vi "MATRIX.vi"() -> ()   [LabVIEW 2012]
uses:
  <vilib>/Instr/_visa.llb/VISA Configure Serial Port (Instr).vi
panel:
  in  "Texte":string
  in  "Afficher":bool
  in  "Effacer":bool
  in  "Défilement 2":bool
  in  "Afficher l'heure":bool
  in  "Envoyer un texte":bool
  out "Array booleano":bool[][](array[boolean])
  in  "Colonnes":u32=30
  in  "Texte d'éssai":string
  in  "Défilement":bool
  in  "Abrir fuente":bool
  in  "Salir":bool
  in  "Vitesse de défilement":dbl(slide)=21.09090909090909 scale=1.0..40.0
  out "chaîne d'heure":string
  out "chaîne de date":string
  out "Date et heure":timestamp format="%<%X\n%x>T"
  in  "COM Port":refnum<visa-resource-name>
  # "Mini Projet 2015"
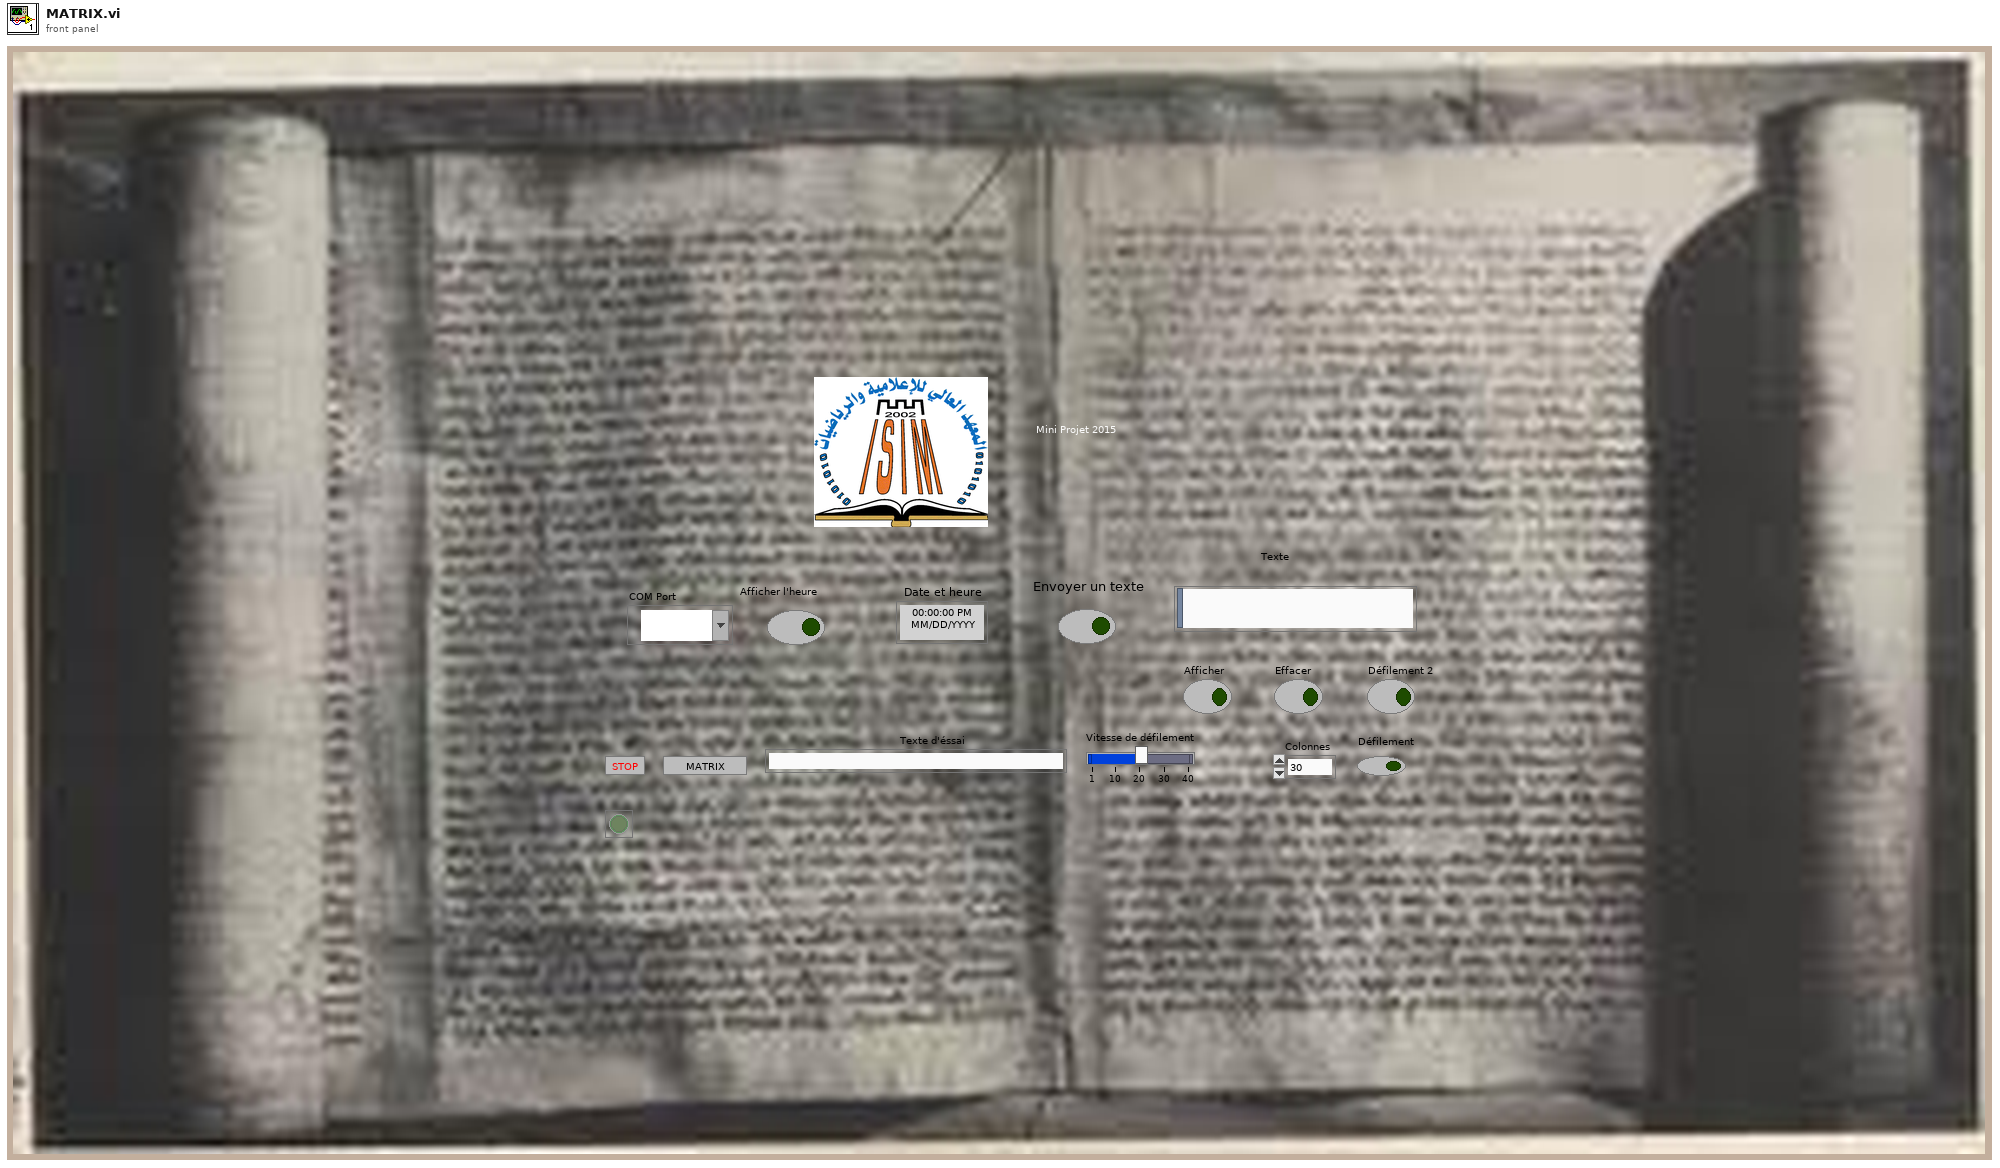
[diagram p1: front panel]
types:
  T1 = enum16{"open", "replace", "create", "open or create", "replace or create", "replace or create with confirmation"}
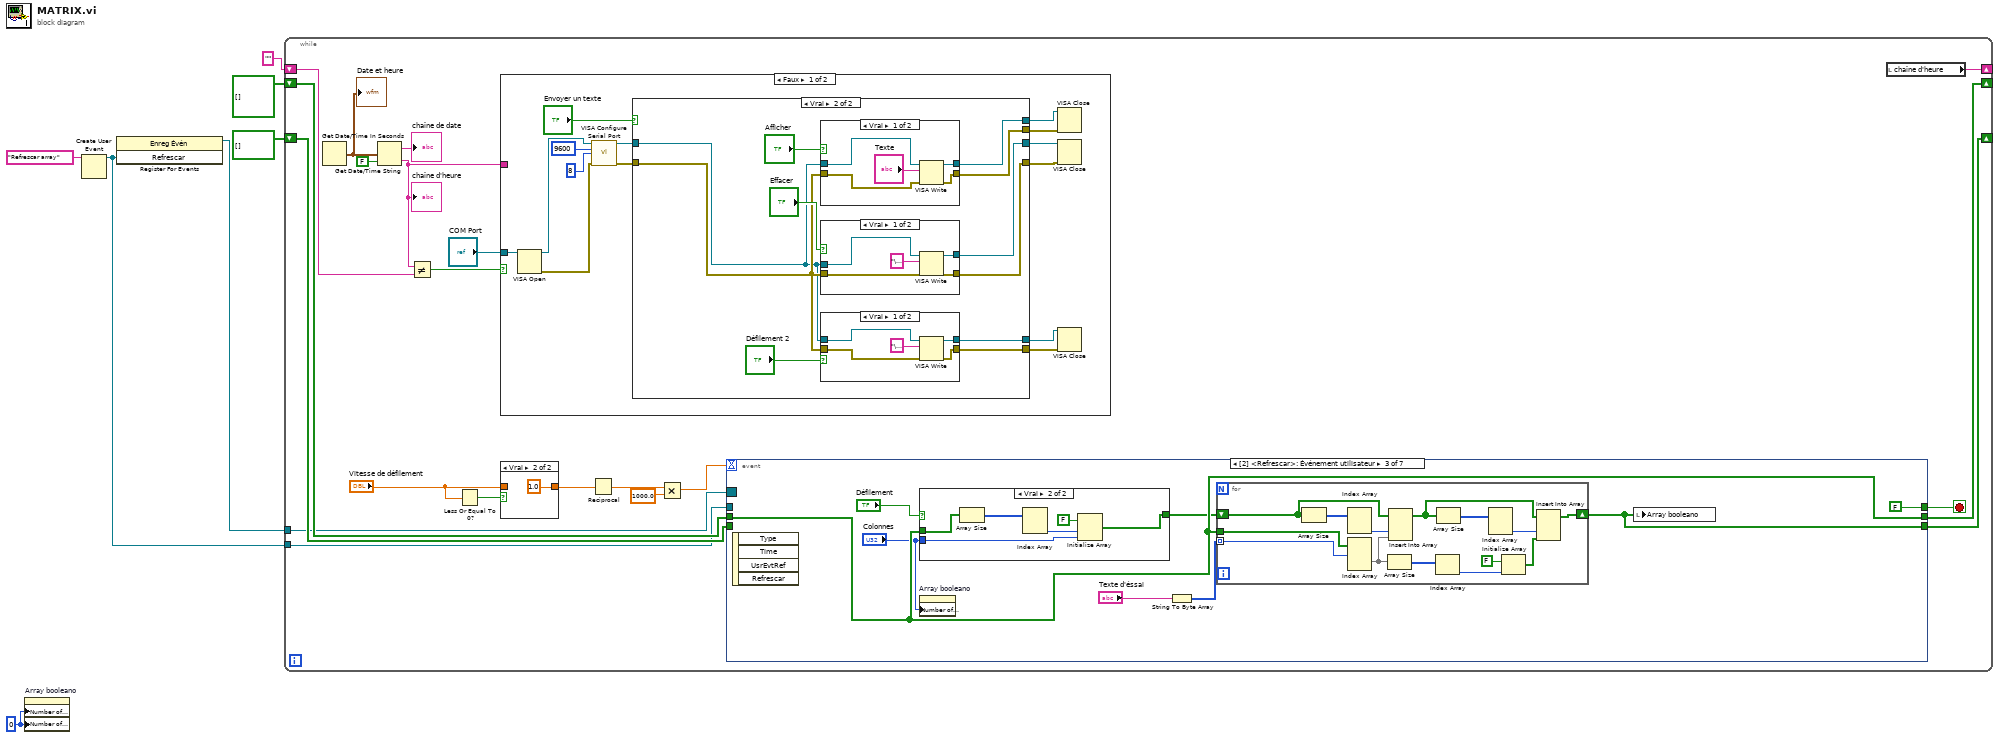
[diagram p0: block diagram]
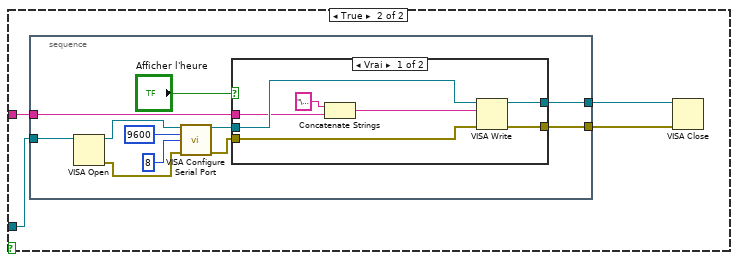
[diagram p6: hidden frame]
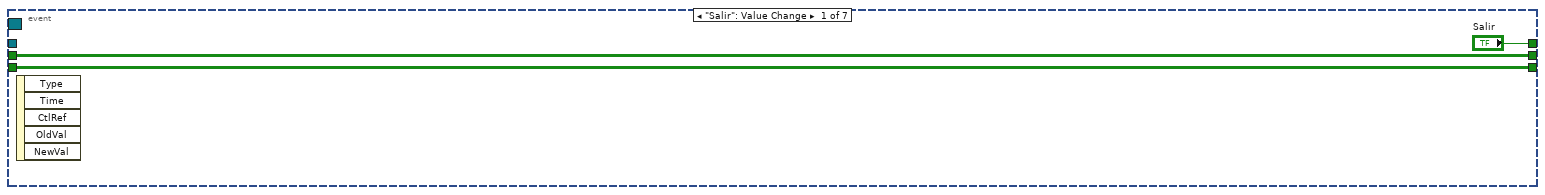
[diagram p9: hidden frame]
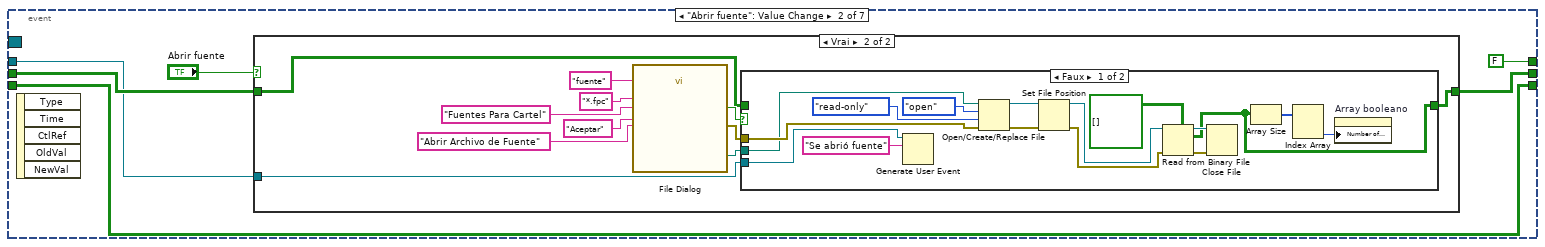
[diagram p10: hidden frame]
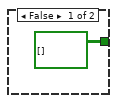
[diagram p13: hidden frame]
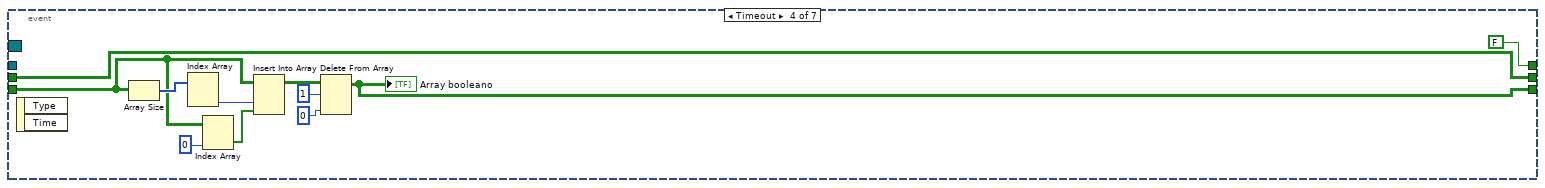
[diagram p14: hidden frame]
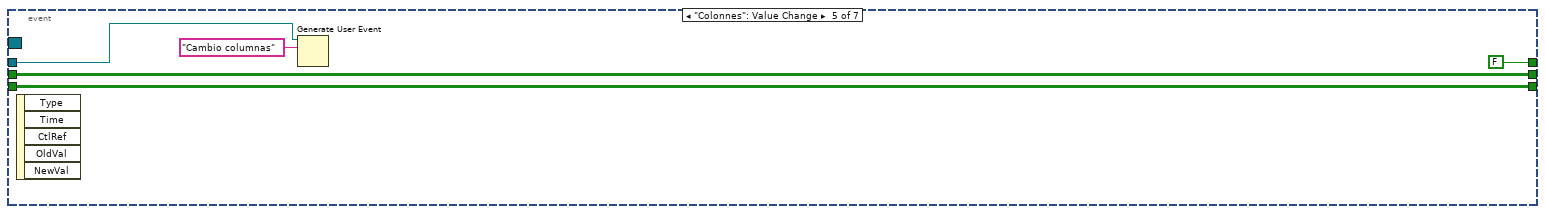
[diagram p15: hidden frame]
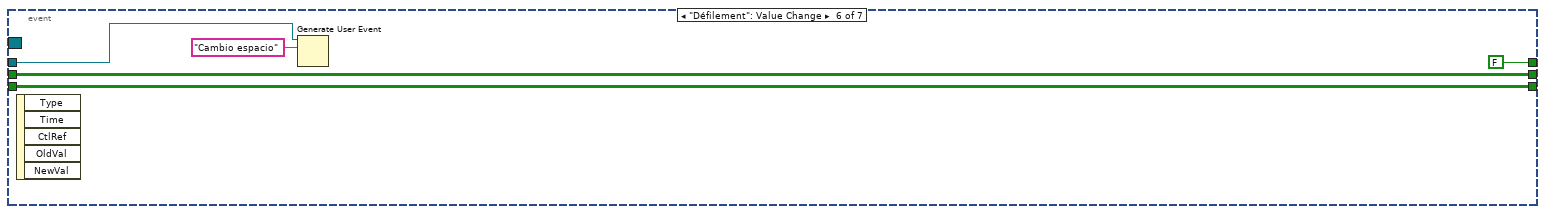
[diagram p16: hidden frame]
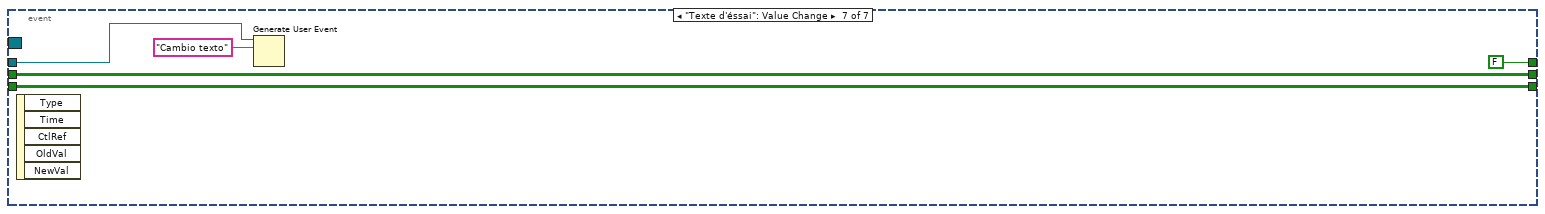
[diagram p17: hidden frame]
diagram:
  w2 = u32 0 ("Number of Columns")
  n1 = property on="Array booleano" class="Tabl (strict)"("Number of Columns"=w2, "Number of Rows"=w2) -> ()  [unwired: 2 in, 2 out]
  n2 = Create User Event(user event datatype="Refrescar array" ("Refrescar")) -> (user event=w3:refnum<user-event>)  [unwired: 1 in, 1 out]
  n3 = register-events(w3) -> (reference out=w4:refnum<event-registration>)  [unwired: 2 in, 1 out]
  n4 = while {
    shift-right: [w20] -> _
    shift-left: bool[][][] [] ("appended array") -> [w19]
    shift-right: [w21] -> _
    shift-left: bool[][] [] ("Array booleano") -> [w18]
    tunnel: w4 -> [w17]
    tunnel: w3 -> [w16]
    shift-right: [w11] -> _
    shift-left: "" ("chaîne d'heure") -> [w9]
    stop <- w15 stop-if-true
    n5 = Get Date/Time In Seconds() -> (seconds since 1Jan1904=w12:timestamp)
    "Date et heure" <- w12
    n6 = Get Date/Time String(seconds (now)=w12, want seconds? (F)=FALSE ("secondes ? (F)")) -> (date string=→"chaîne de date":string, time string=w10:string)  [unwired: 1 in]
    "chaîne d'heure" <- w10
    n7 = Not Equal?(x=w10, y=w9) -> (x != y?=w8:bool)
    n8 = Less Or Equal To 0?(x="Vitesse de défilement") -> (x <= 0?=w24:bool)
    n9 = case shown="Faux" w8 {
      tunnel: "COM Port" -> [w38 w80]
      tunnel: w10 -> [_ w77]
      frame False {
        n10 = VISA Open(VISA resource name=w38) -> (VISA resource name=w40:refnum<visa-resource-name>, error out=w39:errorcluster)  [unwired: 4 in]
        n11 = call-poly "VISA Configure Serial Port"("VISA resource name"=w40, "baud rate (9600)"=u32 9600, "data bits (8)"=u16 8, "error in (no error)"=w39) -> ("VISA resource name out"=w36:refnum<visa-resource-name>, "error out"=w37:errorcluster)  [unwired: 10 in]
        n12 = case shown="Vrai" "Envoyer un texte" {
          tunnel: [w44 w54] -> w30
          tunnel: [w43 w53] -> w29
          tunnel: [w44 w52] -> w32
          tunnel: [w43 w51] -> w31
          tunnel: w37 -> [w43 w48]
          tunnel: w36 -> [w44 w47]
          tunnel: [w44 w46] -> w34
          tunnel: [w43 w45] -> w33
          frame False {
          }
          frame True {
            n13 = case shown="Vrai" "Afficher" {
              tunnel: w48 -> [w74 w75]
              tunnel: w47 -> [w73 w76]
              tunnel: [w72 w76] -> w54
              tunnel: [w71 w75] -> w53
              frame True {
                n14 = VISA Write(VISA resource name=w73, write buffer="Texte", error in (no error)=w74) -> (VISA resource name out=w72:refnum<visa-resource-name>, error out=w71:errorcluster)  [unwired: 1 out]
              }
              frame False {
              }
            }
            n15 = case shown="Vrai" "Effacer" {
              tunnel: w48 -> [w67 w68]
              tunnel: w47 -> [w66 w69]
              tunnel: [w65 w69] -> w52
              tunnel: [w64 w68] -> w51
              frame True {
                n16 = VISA Write(VISA resource name=w66, write buffer="\u0004" ("buffer d'écriture"), error in (no error)=w67) -> (VISA resource name out=w65:refnum<visa-resource-name>, error out=w64:errorcluster)  [unwired: 1 out]
              }
              frame False {
              }
            }
            n17 = case shown="Vrai" "Défilement 2" {
              tunnel: w48 -> [w60 w61]
              tunnel: w47 -> [w59 w62]
              tunnel: [w58 w62] -> w46
              tunnel: [w57 w61] -> w45
              frame True {
                n18 = VISA Write(VISA resource name=w59, write buffer="\u000b" ("buffer d'écriture"), error in (no error)=w60) -> (VISA resource name out=w58:refnum<visa-resource-name>, error out=w57:errorcluster)  [unwired: 1 out]
              }
              frame False {
              }
            }
          }
        }
        n19 = VISA Close(VISA resource name=w30, error in (no error)=w29) -> ()  [unwired: 1 out]
        n20 = VISA Close(VISA resource name=w32, error in (no error)=w31) -> ()  [unwired: 1 out]
        n21 = VISA Close(VISA resource name=w34, error in (no error)=w33) -> ()  [unwired: 1 out]
      }
      frame True {
        n22 = stacked-sequence {
          tunnel: w80 -> [w89]
          tunnel: [w87] -> w79
          tunnel: [w88] -> w78
          tunnel: w77 -> [w82]
          frame #0 {
            n23 = VISA Open(VISA resource name=w89) -> (VISA resource name=w90:refnum<visa-resource-name>, error out=w91:errorcluster)  [unwired: 4 in]
            n24 = call-poly "VISA Configure Serial Port"("VISA resource name"=w90, "baud rate (9600)"=u32 9600, "data bits (8)"=u16 8, "error in (no error)"=w91) -> ("VISA resource name out"=w83:refnum<visa-resource-name>, "error out"=w84:errorcluster)  [unwired: 10 in]
            n25 = case shown="Vrai" "Afficher l'heure" {
              tunnel: w84 -> [w98 w99]
              tunnel: w83 -> [w97 w100]
              tunnel: [w96 w100] -> w88
              tunnel: [w95 w99] -> w87
              tunnel: w82 -> [w94 _]
              frame True {
                n26 = Concatenate Strings("\u0004" ("chaîne"), w94) -> (w93:string)
                n27 = VISA Write(VISA resource name=w97, write buffer=w93, error in (no error)=w98) -> (VISA resource name out=w96:refnum<visa-resource-name>, error out=w95:errorcluster)  [unwired: 1 out]
              }
              frame False {
              }
            }
          }
        }
        n28 = VISA Close(VISA resource name=w78, error in (no error)=w79) -> ()  [unwired: 1 out]
      }
    }
    n29 = case shown="Vrai" w24 {
      tunnel: "Vitesse de défilement" -> [w101 _]
      tunnel: [w101 1.0 ("Velocidad texto [caracteres/segundo]")] -> w25
      frame False {
      }
      frame True {
      }
    }
    n30 = Reciprocal(x=w25) -> (1/x=w26:dbl)
    n31 = Multiply(x=w26, y=1000.0) -> (x*y=w22:dbl)
    n32 = event shown="[2] <Refrescar>: Événement utilisateur" {
      selector: w17 -> [_ _ _ _ _ _ _]
      dyn-events: _ -> [_ _ _ _ _ _ _]
      timeout: w22 -> [_ _ _ _ _ _ _]
      tunnel: ["Salir" FALSE ("Salir") FALSE ("Salir") FALSE ("Salir") FALSE ("Salir") FALSE ("Salir") FALSE ("Salir")] -> w15
      tunnel: w19 -> [w104 w109 w143 w179 w184 w187 w192]
      tunnel: [w104 w108 w143 w179 w184 w187 w192] -> w20
      tunnel: w16 -> [_ w107 _ _ w183 w189 w194]
      tunnel: w18 -> [w103 w106 _ w177 w181 w188 w193]
      tunnel: [w103 w106 w145 w173 w181 w188 w193] -> w21
      event "Salir": Value Change {
        n33 = event-data() -> ()  [unwired: 1 in, 5 out]
      }
      event "Abrir fuente": Value Change {
        n34 = event-data() -> ()  [unwired: 1 in, 5 out]
        n35 = case shown="Vrai" "Abrir fuente" {
          tunnel: [w112 w115] -> w108
          tunnel: w109 -> [w112 w114]
          tunnel: w107 -> [_ w113]
          frame False {
          }
          frame True {
            n36 = call "File Dialog"("prompt"="Abrir Archivo de Fuente", "button label"="Aceptar", "default name"="fuente", "pattern (all files)"="*.fpc", "pattern label"="Fuentes Para Cartel") -> ("selected path"=w116:path, "cancelled"=w118:bool, "error out"=w117:errorcluster)  [unwired: 7 in, 1 out]
            n37 = case shown="Faux" w118 {
              tunnel: w117 -> [w139 _]
              tunnel: w116 -> [w129 _]
              tunnel: [w128 w140] -> w115
              tunnel: w114 -> [_ w140]
              tunnel: w113 -> [w125 _]
              frame False {
                n38 = Generate User Event(user event=w125, event data cluster="Se abrió fuente" ("event data")) -> ()  [unwired: 1 in, 2 out]
                n39 = Open/Create/Replace File(file path (use dialog)=w129, error in=w139, operation (0:open)=T1."open", access (0:read/write)=enum16{"read/write", "read-only", "write-only"}."read-only") -> (refnum out=w135:refnum<file>, error out=w136:errorcluster)  [unwired: 2 in, 1 out]
                n40 = Set File Position(refnum=w135, error in=w136) -> (refnum out=w133:refnum<file>, error out=w134:errorcluster)  [unwired: 2 in]
                n41 = Read from Binary File(5:bool[][][] [] ("appended array"), 8:w134, 11:w133) -> (0:w131:errorcluster, 2:w128:bool[][][], 3:w132:refnum<file>)  [unwired: 3 in, 1 out]
                n42 = Close File(refnum=w132, error in=w131) -> ()  [unwired: 2 out]
                n43 = Array Size(array=w128) -> (size(s)=w127:i32[])
                n44 = Index Array(array=w127) -> (element #2=w126:i32)  [unwired: 2 in, 1 out]
                n45 = property on="Array booleano" class="Tabl (strict)"("Number of Rows"=w126) -> ()  [unwired: 2 in, 2 out]
              }
              frame True {
              }
            }
          }
        }
      }
      event User Event {
        n46 = event-data() -> ()  [unwired: 1 in, 4 out]
        n47 = case shown="Vrai" "Défilement" {
          tunnel: w143 -> [_ w153]
          tunnel: "Colonnes" -> [_ w151]
          tunnel: [bool[][] [] ("Array booleano") w150] -> w141
          frame False {
          }
          frame True {
            n48 = Array Size(array=w153) -> (size(s)=w155:i32[])
            n49 = Index Array(array=w155) -> (element #2=w152:i32)  [unwired: 2 in, 1 out]
            n50 = Initialize Array(FALSE, w152, w151) -> (w150:bool[][])
          }
        }
        n51 = property on="Array booleano" class="Tabl (strict)"("Number of Columns"="Colonnes") -> ()  [unwired: 2 in, 2 out]
        n52 = String To Byte Array(string="Texte d'éssai") -> (unsigned byte array=w146:u8[])
        n53 = for {
          tunnel: w146 -> [w168] mode=indexing
          shift-right: [w163] -> w145
          shift-left: w141 -> [w167]
          tunnel: w143 -> [w169]
          n54 = Array Size(array=w167) -> (size(s)=w166:i32[])
          n55 = Index Array(array=w166) -> (element #2=w156:i32)  [unwired: 2 in, 1 out]
          n56 = Index Array(array=w169, index (dim 0)=w168) -> (element=w162:bool[][])  [unwired: 2 in]
          n57 = Array Size(array=w162) -> (size(s)=w161:i32[])
          n58 = Insert Into Array(array=w167, index (col)=w156, new element=w162) -> (w159:bool[][])  [unwired: 1 in]
          n59 = Index Array(array=w161) -> (element=w160:i32)  [unwired: 1 in]
          n60 = Array Size(array=w159) -> (size(s)=w158:i32[])
          n61 = Index Array(array=w158) -> (element #2=w157:i32)  [unwired: 2 in, 1 out]
          n62 = Initialize Array(FALSE, w160) -> (w164:bool[])
          n63 = Insert Into Array(array=w159, index (col)=w157, new element=w164) -> (w163:bool[][])  [unwired: 1 in]
        }
        n64 = local write "Array booleano"(w145) -> ()
      }
      event Timeout {
        n65 = event-data() -> ()  [unwired: 1 in, 2 out]
        n66 = Array Size(array=w177) -> (size(s)=w178:i32[])
        n67 = Index Array(array=w178) -> (element #2=w171:i32)  [unwired: 2 in, 1 out]
        n68 = Index Array(array=w177, index (col)=0 ("disabled index (col)")) -> (element=w176:bool[])  [unwired: 1 in]
        n69 = Insert Into Array(array=w177, index (col)=w171, new element=w176) -> (w175:bool[][])  [unwired: 1 in]
        n70 = Delete From Array(array=w175, length=1, index (col)=0 ("index (row)")) -> (array with subset deleted=w173:bool[][])  [unwired: 1 in, 1 out]
        "Array booleano" <- w173
      }
      event "Colonnes": Value Change {
        n71 = event-data() -> ()  [unwired: 1 in, 5 out]
        n72 = Generate User Event(user event=w183, event data cluster="Cambio columnas" ("event data")) -> ()  [unwired: 1 in, 2 out]
      }
      event "Défilement": Value Change {
        n73 = event-data() -> ()  [unwired: 1 in, 5 out]
        n74 = Generate User Event(user event=w189, event data cluster="Cambio espacio" ("event data")) -> ()  [unwired: 1 in, 2 out]
      }
      event "Texte d'éssai": Value Change {
        n75 = event-data() -> ()  [unwired: 1 in, 5 out]
        n76 = Generate User Event(user event=w194, event data cluster="Cambio texto" ("event data")) -> ()  [unwired: 1 in, 2 out]
      }
    }
    n77 = local read "chaîne d'heure"() -> (w11:string)
  }
